vi "asdk Get.vi"(8 "error in (no error)":errorcluster, 10 "command":string, 11 "pDm":u64) -> (0 "error out":errorcluster, 1 "value out":dbl, 3 "pDm out":u64)   [LabVIEW 2020, in "ASDK.lvlib"]
doc: "ASDK_API COMPL_STAT asdkGet( asdkDM *pDm, CStrConst command, Scalar * value );"
uses:
  ASDK.lvlib
  ASDK.dll
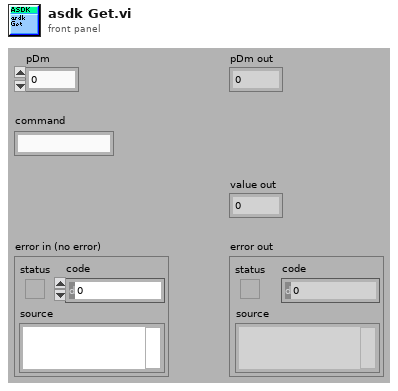
[diagram p1: front panel]
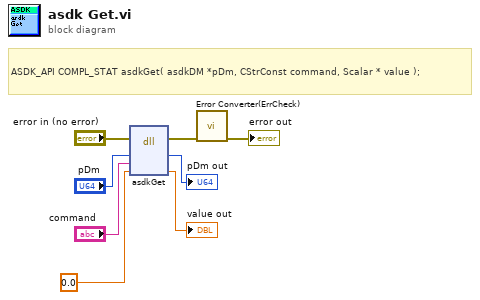
[diagram p0: block diagram]
diagram:
  # "ASDK_API COMPL_STAT asdkGet( asdkDM *pDm, CStrConst command, Scalar * value );"
  n1 = dll-call lib="ASDK.*" fn="asdkGet"(error in="error in (no error)", "pDm"="pDm", "command"="command", "value"=0.0) -> (error out=w3:errorcluster, "pDm"=→"pDm out":u64, "value"=→"value out":dbl)  [unwired: 4 in, 1 out]
  n2 = call "Error Converter(ErrCheck).vi"("error in (no error)"=w3) -> ("error out"=→"error out":errorcluster)  [unwired: 10 in]
